vi "ADC Example (A).vi"() -> ()   [LabVIEW 2011]
doc: "Advanced Analog Digital Converter"
uses:
  C:/Program Files/Metrohm Autolab/Autolab SDK 1.10/EcoChemie.Autolab.Sdk.dll
  EcoChemie.Autolab.Sdk.dll
panel:
  in  "Channel":i32(ring) items=["16"=15, "15"=14, "14"=13, "13"=12, "12"=11, "11"=10, "10"=9, "9"=8, "8"=7, "7"=6, "6"=5, "5"=4, "4"=3, "3"=2, "2"=1, "1"=0]
  out "Sample":dbl
  in  "usPerLoop 2":u16=20000
  in  "usPerLoop":u16=20000
  in  "Sampler Type":T1(ring)
  in  "Loops 2":i32=1 min=1
  in  "Loops":i32=1 min=1
  in  "Gain 2":i32(ring) items=["Gain_1"=0, "Gain_10"=64, "Gain_100"=128, "Gain_1000"=192]
  in  "Gain":i32(ring) items=["Gain_1"=0, "Gain_10"=64, "Gain_100"=128, "Gain_1000"=192]
  out "error out":errorcluster
  in  "stop":bool
  out "IsConnected":bool
  in  "Hardware Setup File":path
  in  "Embedded Exe File":path
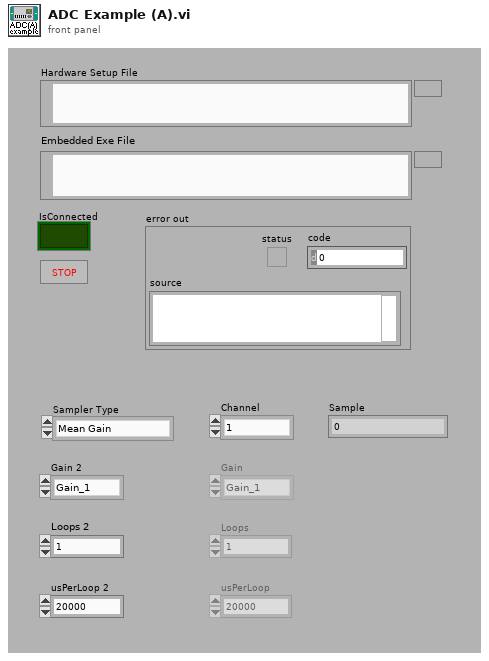
[diagram p1: front panel]
types:
  T1 = enum16{"Mean Gain", "Mean Fixed", "One Fixed", "One Gain"}
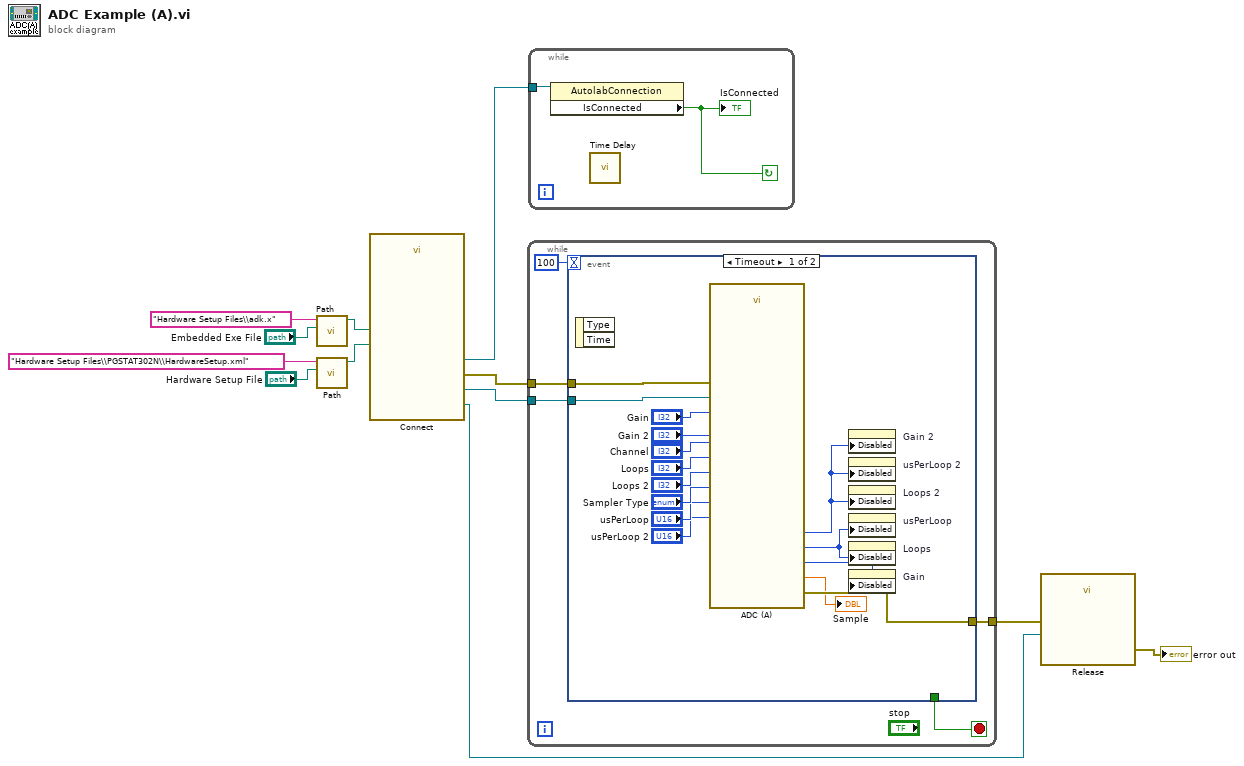
[diagram p0: block diagram]
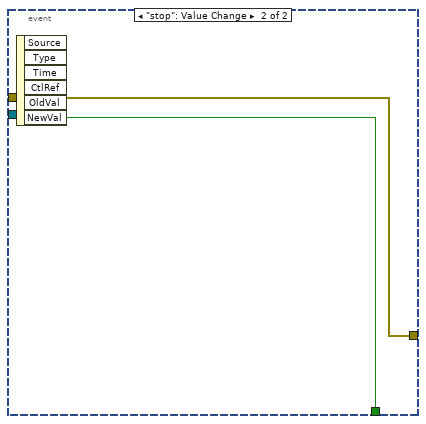
[diagram p2: hidden frame]
diagram:
  n1 = call "Path.vi"("File"="Embedded Exe File", "name or relative path"="Hardware Setup Files\\adk.x") -> ("appended path"=w3:path)  [unwired: 9 in]
  n2 = call "Path.vi"("File"="Hardware Setup File", "name or relative path"="Hardware Setup Files\\PGSTAT302N\\HardwareSetup.xml") -> ("appended path"=w4:path)  [unwired: 9 in]
  n3 = call "Connect.vi"("Embedded Exe File"=w3, "Hardware Setup File"=w4) -> ("Adc"=w9:refnum<k24>, "AutolabConnection"=w8:refnum<k24>, "instrument"=w7:refnum<k24>, "error out"=w10:errorcluster)  [unwired: 6 in, 4 out]
  n4 = while {
    tunnel: w10 -> [w16]
    tunnel: w9 -> [w15]
    tunnel: [w17] -> w11
    stop <- w13 stop-if-true
    n5 = event shown="[0] Timeout" {
      selector: _ -> [_ _]
      dyn-events: _ -> [_ _]
      timeout: 100 -> [_ _]
      tunnel: [w32 w33] -> w17
      tunnel: w16 -> [w31 w33]
      tunnel: w15 -> [w30 _]
      tunnel: [_ w34] -> w13
      event Timeout {
        n6 = event-data() -> ()  [unwired: 1 in, 2 out]
        n7 = call "ADC (A).vi"("Adc"=w30, "Loops 2"="Loops 2", "Gain"="Gain", "Loops"="Loops", "Sampler Type"="Sampler Type", "Gain 2"="Gain 2", "usPerLoop 2"="usPerLoop 2", "error in"=w31, "Channel"="Channel", "usPerLoop"="usPerLoop") -> ("Sample"=→"Sample":dbl, "Disable MeanGain"=w29:u8, "Disable MeanFixed"=w27:u8, "Disable OneFixed"=w28:u8, "error out"=w32:errorcluster)  [unwired: 1 in]
        n8 = property on="Gain 2" class="Ring (strict)"("Disabled"=w27) -> ()  [unwired: 2 in, 2 out]
        n9 = property on="usPerLoop 2" class="DigNum (strict)"("Disabled"=w27) -> ()  [unwired: 2 in, 2 out]
        n10 = property on="Loops 2" class="DigNum (strict)"("Disabled"=w27) -> ()  [unwired: 2 in, 2 out]
        n11 = property on="usPerLoop" class="DigNum (strict)"("Disabled"=w29) -> ()  [unwired: 2 in, 2 out]
        n12 = property on="Loops" class="DigNum (strict)"("Disabled"=w29) -> ()  [unwired: 2 in, 2 out]
        n13 = property on="Gain" class="Ring (strict)"("Disabled"=w28) -> ()  [unwired: 2 in, 2 out]
      }
      event "stop": Value Change {
        n14 = event-data() -> ("NewVal"=w34:bool)  [unwired: 1 in, 5 out]
      }
    }
  }
  n15 = while {
    tunnel: w8 -> [w36]
    stop <- w35 continue-if-true
    n16 = property class="AutolabConnection"(reference=w36) -> ("IsConnected"=w35:bool)  [unwired: 1 in, 2 out]
    "IsConnected" <- w35
    n17 = call "Time Delay"() -> ()  [unwired: 11 in, 1 out]
  }
  n18 = call "Release.vi"("error in (no error)"=w11, "Instrument"=w7) -> ("error out"=→"error out":errorcluster)  [unwired: 9 in]
